vi "Engine - Copy & Script Templates.vi"(8 "error in (no error)":errorcluster, 9 "RT Driver VI Path":path, 10 "RT Driver Folder Path":path, 11 "CD Source Folder Path":path) -> (0 "error out":errorcluster)   [LabVIEW 2015]
doc: "Via scripting, replace the tempate RTStateVariables control with the new type def across the async and RT driver VIs, and script the compiled settings property into the constants global"
uses:
  Constants/Constants TypDef/Common.ctl
  <vilib>/Utility/traverseref.llb/TRef TravTarget.ctl
  Constants/Constants TypDef/CD Engine lvlib.ctl
  Constants/Constants TypDef/CD Shared lvlib.ctl
  Constants/CD Engine lvlib.vi
  Constants/Common.vi
  Constants/CD Shared lvlib.vi
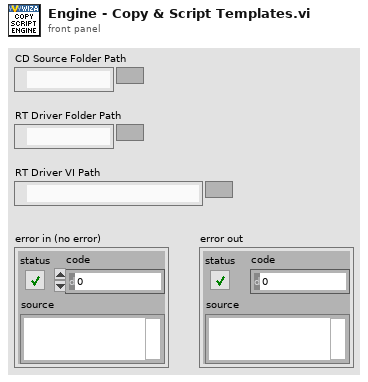
[diagram p1: front panel]
types:
  T1 = typedef "CD Engine lvlib.ctl" = enum16{"LibraryFileName", "LibraryFolderName", "Engine.FolderName", "Engine.Init.FolderName", "Engine.Run.FolderName", "Engine.Shutdown.FolderName", "Types.FolderName", "Engine.RT Driver VI.TemplatePath", "Engine.RT Driver VI.FileName", "Engine.RTStateVariables.Name", "Engine.RTStateVariables.Name.NoExtension", "Engine.Async.NameExtension", "Engine.Async.TemplateName"}
  T2 = typedef "CD Shared lvlib.ctl" = enum16{"LibraryFileName", "LibraryFolderName", "ConstantsVI.VIPathAndName", "Shared.FolderName", "Shared.Types.FolderName", "Shared.Constants.VIName", "Shared.Constants.VITemplateName", "Shared.Constants.VITemplatePathAndName", "Shared.CompiledSettings.RelativePath", "Shared.Constants.RelativePath", "Shared.CompiledSettings.Name", "Shared.CompiledSettings.Name.NoExtension", "Shared.CompiledSettings.ClusterName"}
  T3 = typedef "TRef TravTarget.ctl" = enum16{"FP", "BD", "Other"}
  T4 = typedef "Common.ctl" = enum16{"ProjectName", "TemplatesFolderName", "ProjectTemplatePathAndName", "ReadmeTemplatePathAndName", "TimingAndSyncFolderName", "CustomDeviceFolderName", "PathToTemplates"}
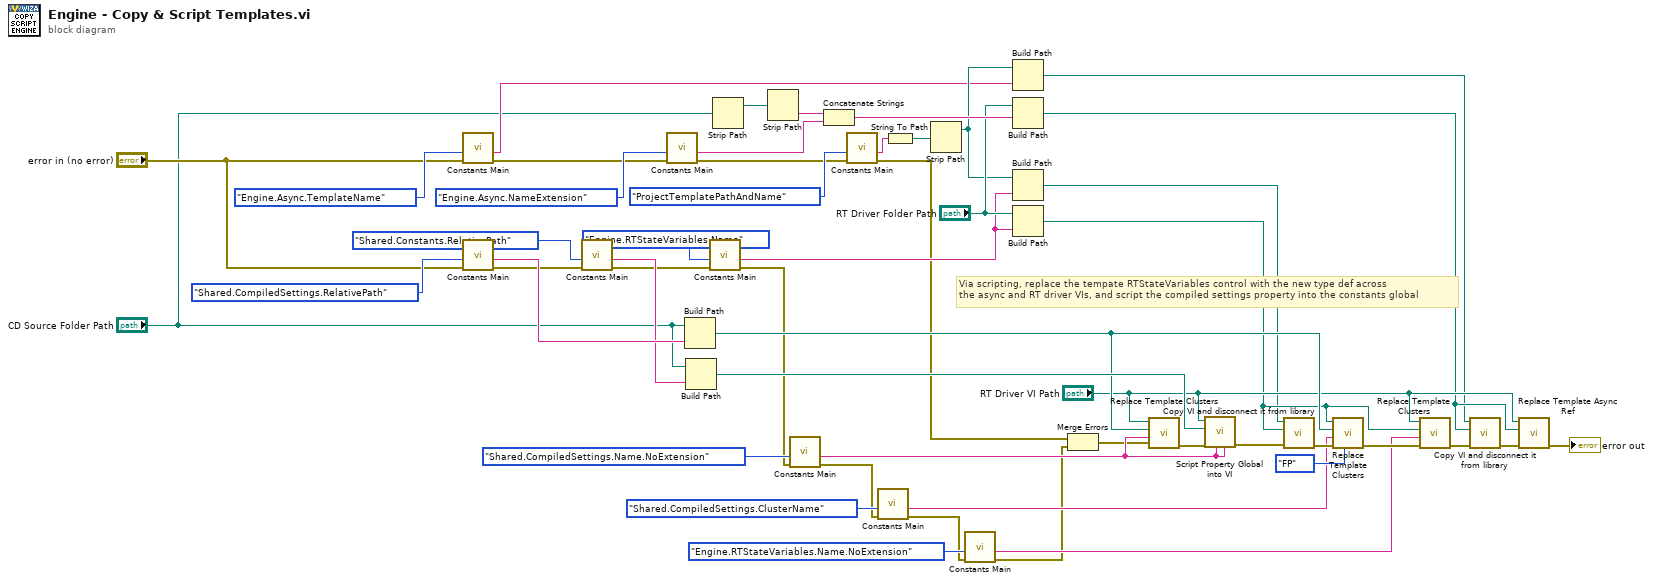
[diagram p0: block diagram]
diagram:
  # "Via scripting, replace the tempate RTStateVariables control with the new type def across\nthe async and RT driver VIs, and script the compiled settings property into the constants global"
  n1 = call-poly "Constants Main.vi"("error in (no error)"="error in (no error)", "Action"=CD_Engine_lvlib."Engine.Async.TemplateName") -> ("error out"=w25:errorcluster, "Output"=w23:string)  [unwired: 8 in]
  n2 = call-poly "Constants Main.vi"("error in (no error)"="error in (no error)", "Action"=CD_Shared_lvlib."Shared.CompiledSettings.RelativePath") -> ("error out"=w19:errorcluster, "Output"=w20:string)  [unwired: 8 in]
  n3 = call-poly "Constants Main.vi"("error in (no error)"=w19, "Action"=CD_Shared_lvlib."Shared.Constants.RelativePath") -> ("error out"=w14:errorcluster, "Output"=w17:string)  [unwired: 8 in]
  n4 = call-poly "Constants Main.vi"("error in (no error)"=w25, "Action"=CD_Engine_lvlib."Engine.Async.NameExtension") -> ("error out"=w24:errorcluster, "Output"=w27:string)  [unwired: 8 in]
  n5 = Build Path(base path="CD Source Folder Path", name or relative path=w20) -> (appended path=w50:path)
  n6 = Build Path(base path="CD Source Folder Path", name or relative path=w17) -> (appended path=w51:path)
  n7 = call-poly "Constants Main.vi"("error in (no error)"=w14, "Action"=CD_Engine_lvlib."Engine.RTStateVariables.Name") -> ("error out"=w10:errorcluster, "Output"=w13:string)  [unwired: 8 in]
  n8 = Strip Path(path="CD Source Folder Path") -> (stripped path=w41:path)  [unwired: 1 out]
  n9 = Strip Path(path=w41) -> (name=w42:string)  [unwired: 1 out]
  n10 = call-poly "Constants Main.vi"("error in (no error)"=w10, "Action"=CD_Shared_lvlib."Shared.CompiledSettings.Name.NoExtension") -> ("error out"=w8:errorcluster, "Output"=w11:string)  [unwired: 8 in]
  n11 = Concatenate Strings(w42, w27) -> (w43:string)
  n12 = call-poly "Constants Main.vi"("error in (no error)"=w24, "Action"=Common."ProjectTemplatePathAndName") -> ("error out"=w3:errorcluster, "Output"=w30:string)  [unwired: 8 in]
  n13 = call-poly "Constants Main.vi"("error in (no error)"=w8, "Action"=CD_Shared_lvlib."Shared.CompiledSettings.ClusterName") -> ("error out"=w4:errorcluster, "Output"=w7:string)  [unwired: 8 in]
  n14 = String To Path(string=w30) -> (path=w31:path)
  n15 = Strip Path(path=w31) -> (stripped path=w37:path)  [unwired: 1 out]
  n16 = call-poly "Constants Main.vi"("error in (no error)"=w4, "Action"=CD_Engine_lvlib."Engine.RTStateVariables.Name.NoExtension") -> ("error out"=w2:errorcluster, "Output"=w5:string)  [unwired: 8 in]
  n17 = Build Path(base path=w37, name or relative path=w23) -> (appended path=w40:path)
  n18 = Build Path(base path="RT Driver Folder Path", name or relative path=w43) -> (appended path=w46:path)
  n19 = Build Path(base path=w37, name or relative path=w13) -> (appended path=w32:path)
  n20 = Build Path(base path="RT Driver Folder Path", name or relative path=w13) -> (appended path=w36:path)
  n21 = Merge Errors(w3, w2) -> (w1:errorcluster)
  n22 = call "Replace Template Clusters.vi"("error in (no error)"=w1, "Control Name"=w11, "Path to Cluster to Replace"=w50, "Path to VI"="RT Driver VI Path") -> ("error out"=w47:errorcluster)  [unwired: 7 in]
  n23 = call "Script Property Global into VI.vi"("GlobalControlName"=w11, "StringConstantToReplace"=w11, "error in (no error)"=w47, "Path to Global"=w51, "Path to VI"="RT Driver VI Path") -> ("error out"=w48:errorcluster)  [unwired: 6 in]
  n24 = call "Copy VI and disconnect it from library.vi"("error in (no error)"=w48, "VI Target Path"=w36, "VI Source Path"=w32) -> ("error out"=w33:errorcluster)  [unwired: 8 in]
  n25 = call "Replace Template Clusters.vi"("Traverse Target"=TRef_TravTarget."FP", "error in (no error)"=w33, "Control Name"=w7, "Path to Cluster to Replace"=w50, "Path to VI"=w36) -> ("error out"=w35:errorcluster)  [unwired: 6 in]
  n26 = call "Replace Template Clusters.vi"("error in (no error)"=w35, "Control Name"=w5, "Path to Cluster to Replace"=w36, "Path to VI"="RT Driver VI Path") -> ("error out"=w39:errorcluster)  [unwired: 7 in]
  n27 = call "Copy VI and disconnect it from library.vi"("error in (no error)"=w39, "VI Target Path"=w46, "VI Source Path"=w40) -> ("error out"=w44:errorcluster)  [unwired: 8 in]
  n28 = call "Replace Template Async Ref.vi"("error in (no error)"=w44, "Path to Desired Async VI"=w46, "Path to RT Driver VI"="RT Driver VI Path") -> ("error out"=→"error out":errorcluster)  [unwired: 8 in]
